vi "Configure Measurement Edge (Delay).vi"(5 "Edge Occurrence 2  (1)":i32=1, 7 "Edge Slope 2 (0: Positive)":i32(ring) items=["Positive", "Negative"], 8 "error in (no error)":errorcluster, 9 "Edge Occurrence 1  (1)":i32=1, 10 "Edge Slope 1 (0: Positive)":i32(ring) items=["Positive", "Negative"], 11 "VISA resource name":refnum<visa-resource-name>) -> (0 "error out":errorcluster, 3 "VISA resource name out":refnum<visa-resource-name>)   [LabVIEW 2015, in "Agilent 2000 3000 X-Series.lvlib"]
doc: "Configure the edge definition for delay in measurement."
uses:
  Agilent 2000 3000 X-Series.lvlib
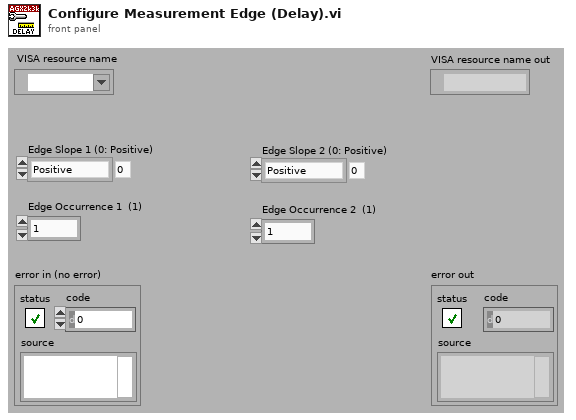
[diagram p1: front panel]
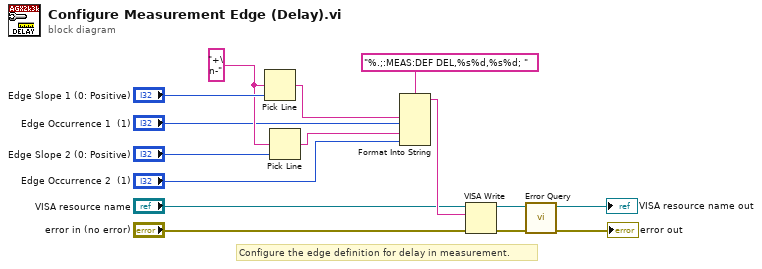
[diagram p0: block diagram]
diagram:
  w13 = "+\n-"
  # "Configure the edge definition for delay in measurement."
  n1 = Pick Line(multi-line string=w13, line index="Edge Slope 1 (0: Positive)") -> (output string=w8:string)  [unwired: 1 out]
  n2 = Pick Line(multi-line string=w13, line index="Edge Slope 2 (0: Positive)") -> (output string=w10:string)  [unwired: 1 out]
  n3 = Format Into String(format string="%.;:MEAS:DEF DEL,%s%d,%s%d; ", w8, "Edge Occurrence 1  (1)", w10, "Edge Occurrence 2  (1)") -> (resulting string=w7:string)  [unwired: 2 in, 1 out]
  n4 = VISA Write(VISA resource name="VISA resource name", write buffer=w7, error in (no error)="error in (no error)") -> (VISA resource name out=w4:refnum<visa-resource-name>, error out=w3:errorcluster)  [unwired: 1 out]
  n5 = call "Error Query.vi"("error in (no error)"=w3, "VISA resource name"=w4) -> ("error out"=→"error out":errorcluster, "VISA resource name out"=→"VISA resource name out":refnum<visa-resource-name>)  [unwired: 8 out]
